vi "Line 1 to End Switch 1.vi"(6 "Command Info In":T3, 8 "Line1 to ESwitch1":T2={"Forward Distance"=130.0, " Forward Speed"=1.0, "Turn Angle"=90.0, "Switch Distance"=20.0, "Switch Speed"=0.5}, 9 "Position":T1=enum."Far Right") -> (0 "Command Info Out":T3)   [LabVIEW 2017]
uses:
  <vilib>/Rock Robotics/WPI/Framework/Command Status Info.ctl
  <vilib>/Rock Robotics/WPI/Framework/Completion Status.ctl
  <vilib>/Rock Robotics/WPI/Framework/Completion Notifier.ctl
  Block Clusters/Line1 to ESwitch1.ctl
  Support Code/Starting Position.ctl
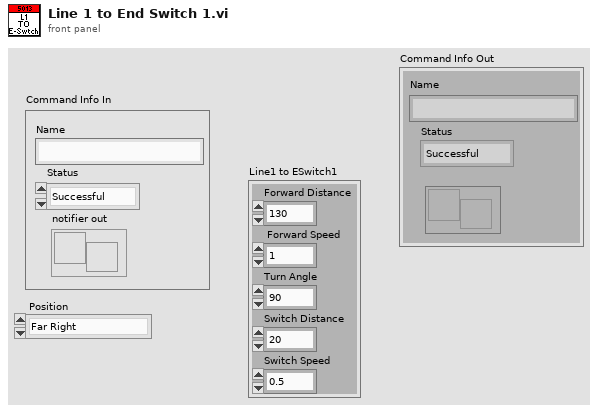
[diagram p1: front panel]
types:
  T1 = typedef "Starting Position.ctl" = enum16{"Far Left", "Center", "Far Right"}
  T2 = typedef "Line1 to ESwitch1.ctl" = cluster{"Forward Distance":dbl, " Forward Speed":dbl, "Turn Angle":dbl, "Switch Distance":dbl, "Switch Speed":dbl}
  T3 = typedef "Command Status Info.ctl" = cluster{"Name":string, "Status":T4, "notifier out":T5}
  T4 = typedef "Completion Status.ctl" = enum16{"Successful", "Aborted", "Incomplete"}
  T5 = typedef "Completion Notifier.ctl" = refnum<notifier>
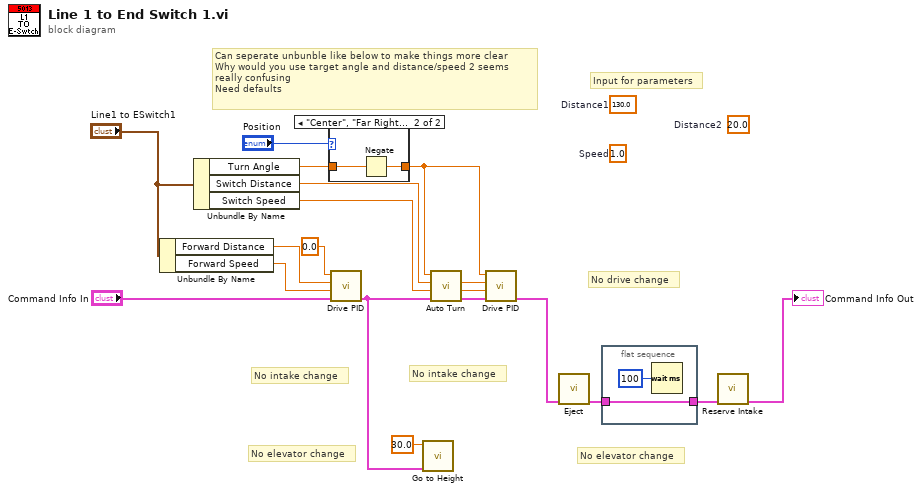
[diagram p0: block diagram]
diagram:
  (unwired) 20.0  # Distance2
  (unwired) 1.0  # Speed
  (unwired) 130.0  # Distance1
  # "Can seperate unbunble like below to make things more clear\nWhy would you use target angle and distance/speed 2 seems\nreally confusing\nNeed defaults"
  # "Input for parameters"
  # "No drive change"
  # "No elevator change"
  # "No intake change"
  # "No intake change"
  # "No elevator change"
  n1 = Unbundle By Name("Line1 to ESwitch1") -> ("Forward Distance"=w4:dbl, "Forward Speed"=w3:dbl)
  n2 = Unbundle By Name("Line1 to ESwitch1") -> ("Turn Angle"=w10:dbl, "Switch Distance"=w6:dbl, "Switch Speed"=w5:dbl)
  n3 = case shown="\"Center\", \"Far Right\"" "Position" {
    tunnel: [w18 w20] -> w11
    tunnel: w10 -> [w18 w19]
    frame "Far Left", Default {
    }
    frame "Center", "Far Right" {
      n4 = Negate(x=w19) -> (-x=w20:dbl)
    }
  }
  n5 = call "Drive PID.vi"("Command Info In"="Command Info In", "Speed"=w3, "Distance"=w4, "Target Angle"=0.0 ("Distance")) -> ("Command Info Out"=w13:T3)  [unwired: 7 in]
  n6 = call "Go to Height.vi"("Command Info In"=w13, "Target Height (in)"=30.0) -> ()  [unwired: 9 in, 1 out]
  n7 = call "Auto Turn.vi"("Command Info In"=w13, "Target Angle"=w11) -> ("Command Info Out"=w14:T3)  [unwired: 9 in]
  n8 = call "Drive PID.vi"("Command Info In"=w14, "Speed"=w5, "Distance"=w6, "Target Angle"=w11) -> ("Command Info Out"=w15:T3)  [unwired: 7 in]
  n9 = call "Eject.vi"("Command Info In"=w15) -> ("Command Info Out"=w16:T3)  [unwired: 10 in]
  n10 = flat-sequence {
    tunnel: w16 -> [w22]
    tunnel: [w22] -> w12
    frame #0 {
      n11 = Wait (ms)(milliseconds to wait=u32 100) -> ()  [unwired: 1 out]
    }
  }
  n12 = call "Reserve Intake.vi"("Command Info"=w12) -> ("Command Info"=→"Command Info Out":T3)  [unwired: 10 in]
